vi "ImagingEventStream-SimpleFifoImage.vi"() -> ()   [LabVIEW 2017]
doc: "This example demonstrates how to use the Becker&Hickl LabVIEW wrapper VIs to acquire a single image in Fifo-Imaging mode.\nThe Event Data is interpreted and populates a 4D DecayMatrix which is then saved as SDT-file to disc.\n\ninfo@becker.hickl.com"
uses:
  SPC_Wrappers/SPC_Controls/SPCdata.ctl
  SPC_Wrappers/SPC_Controls/SPC_RatesCluster.ctl
  Example_Controls/UserInput.ctl
  SPC_Wrappers/SPC_Controls/StateCluster.ctl
  SPC_Wrappers/SPC_Controls/dither_range.ctl
  SPC_Wrappers/Initialisation/SPC_get_error_string.vi
panel:
  out "Overflow, Stop":bool
  out "DecayMatrix":u16[][][][](array[numeric])
  in  "Abort":bool
  in  "include Intensity Image":bool=TRUE
  out "SPC_StateCluster":T1
  in  "User Input":T2={"tac_range"=50.033573, "tac_gain"=2, "tac_offset"=5.0, "tac_limit_high"=89.803925, "tac_limit_low"=10.196078, "collect_time"=10.0, "sync_threshold"=-71.0, "sync_zc_level"=-5.2999988, "sync_freq_div"=1, "cfd_limit_low"=-50.0, "cfd_zc_level"=5.3000016} {"sync_freq_div" items=["1"=1, "2"=2, "4"=4]; "cfd_zc_level" min=-96 max=96 step=0.1 format="%#_3g"; "cfd_limit_low" min=-500 max=0 step=0.1 format="%#_3g"; "sync_zc_level" min=-96 max=96 step=0.1 format="%#_3g"; "sync_threshold" min=-500 max=-20 step=0.1 format="%#_3g"; "tac_limit_low" format="%.3g"; "tac_limit_high" min=0 max=100 step=0.1 format="%.3g"; "collect_time" min=1e-07 max=100000 step=0.001; "tac_offset" min=0 max=100 step=0.1 format="%.4g"; "tac_gain" min=1 max=15 step=1; "tac_range" format="%^#_6g"}
  out "Photon Count":u64
  in  "NoOfRoutingChannels":u32=1 min=1 max=128 step=1
  out "IntensityImage":u32[][](graph)
  in  "ActiveModule":i32[](listbox)
  out "Curent Read Count":u32 step=1
  in  "SDT-File Path":path=path "C:/temp/test.sdt"
  out "MT clock [ns]":i32=25
  out "AquiredPxEvents":cluster{"X":i32, "Y":i32}
  out "SumOfDecays":u32[](graph)=[0, 0, 0, 0, 0, 0, 0, 0, 0, 0, 0, 0, 0, 0, 0, 0, 0, 0, 0, 0, 0, 0, 0, 0, 0, 0, 0, 0, 0, 0, 0, 0, 0, 0, 0, 0, 0, 0, 0, 0, 0, 0, 0, 0, 0, 0, 0, 0, 0, 0, 0, 0, 0, 0, 0, 0, 0, 0, 0, 0, 0, 0, 0, 0, 0, 0, 0, 0, 0, 0, 0, 0, 0, 0, 0, 0, 0, 0, 0, 0, 0, 0, 0, 0, 0, 6, 125, 109, 110, 121, 134, 1104, 3322, 4416, 4644, 4252, 3880, 3585, 3338, 3099, 2923, 2680, 2526, 2363, 2302, 2065, 2037, 1850, 1835, 1680, 1618, 1495, 1415, 1340, 1354, 1344, 1230, 1205, 1110, 1099, 1055, 1073, 969, 897, 915, 879, 826, 828, 779, 761, 760, 741, 674, 666, 635, 675, 612, 654, 541, 599, 580, 511, 492, 520, 489, 482, 463, 436, 481, 442, 415, 420, 393, 409, 416, 362, 382, 349, 345, 338, 324, 324, 344, 328, 286, 322, 307, 275, 277, 289, 241, 289, 239, 239, 269, 257, 232, 198, 222, 228, 222, 226, 207, 188, 224, 205, 227, 178, 188, 200, 177, 158, 177, 188, 171, 179, 168, 156, 146, 163, 146, 163, 146, 123, 140, 157, 149, 116, 145, 112, 132, 122, 149, 92, 0, 0, 0, 0, 0, 0, 0, 0, 0, 0, 0, 0, 0, 0, 0, 0, 0, 0, 0, 0, 0, 0, 0, 0, 0, 0, 0, 0, 0, 0, 0, 0, 0, 0, 0, 0, 0, 0, 0, 0, 0, 0]
  out "DLL Path":path=path "C:/Program Files (x86)/BH/SPCM/DLL/spcm64.dll"
  out "Clock Status":T3={"Frame Clock"=TRUE, "Line Clock"=TRUE, "Pixel Clock"=TRUE}
  out "SPC_RatesCluster":T4 {"Sync" scale=0.0..6000000.0; "ADC" scale=0.0..1000000.0; "TAC" scale=0.0..1000000.0; "CFD" scale=0.0..1000000.0}
  out "SPCdata":T5={"base_adr"=52672, "init"=0, "cfd_limit_low"=-0.0, "cfd_limit_high"=5.019608, "cfd_zc_level"=-5.2913384, "cfd_holdoff"=5.0, "sync_zc_level"=-5.2913384, "sync_holdoff"=4.0, "sync_threshold"=-70.588234, "tac_range"=50.033573, "sync_freq_div"=1, "tac_gain"=1, "tac_offset"=5.098039, "tac_limit_low"=0.0, "tac_limit_high"=100.0, "adc_resolution"=12, "ext_latch_delay"=0, "collect_time"=1.0, "display_time"=1.0, "repeat_time"=10.0, "stop_on_time"=1, "stop_on_ovfl"=1, "dither_range"=128, "count_incr"=1, "mem_bank"=0, "dead_time_comp"=0, "scan_control"=0, "routing_mode"=0, "tac_enable_hold"=0.0, "pci_card_no"=-1, "mode"=5, "scan_size_x"=1, "scan_size_y"=1, "scan_rout_x"=1, "scan_rout_y"=1, "scan_flyback"=65537, "scan_borders"=0, "scan_polarity"=0, "pixel_clock"=1, "line_compression"=1, "trigger"=0, "pixel_time"=1e-07, "ext_pixclk_div"=1, "rate_count_time"=1.0, "macro_time_clk"=0, "add_select"=0, "test_eep"=1, "adc_zoom"=0, "img_size_x"=1, "img_size_y"=1, "img_rout_x"=1, "img_rout_y"=1, "xy_gain"=1, "master_clock"=0, "adc_sample_delay"=0, "detector_type"=1, "chan_enable"=4191231, "chan_slope"=0, "chan_spec_no"=34835, "tdc_control"=0, "tdc_offset1"=0.0, "tdc_offset2"=0.0, "tdc_offset3"=0.0, "tdc_offset4"=0.0, "tdc_offset5"=0.0, "tdc_offset6"=0.0, "cfd_th5_tdc"=0.0, "cfd_th6_tdc"=0.0, "cfd_zc5_tdc"=0.0, "cfd_zc6_tdc"=0.0, "future_reserve1"=0, "future_reserve2"=0, "future_reserve3"=0, "future_reserve4"=0} {"scan_flyback" format="%x"}
  # "This example demonstrates how to use the Becker&Hickl LabVIEW wrapper VIs to acquire a single image in Fifo-Imaging mode.\nThe Event Data is interpreted and populates a 4D DecayMatrix which is then saved as SDT-file to disc."
  # "See Tip-Strip for details"
  # "TAC / Time Range"
  # "CFD"
  # "(start)"
  # "SYNC"
  # "(stop)"
  # "range"
  # "gain"
  # "threshold(LL)"
  # "offset"
  # "limit high"
  # "limit low"
  # "zero cross(ZC)"
  # "Collection Time"
  # "(c) 2022 Becker & Hickl GmbH\n     ALL RIGHTS RESERVED."
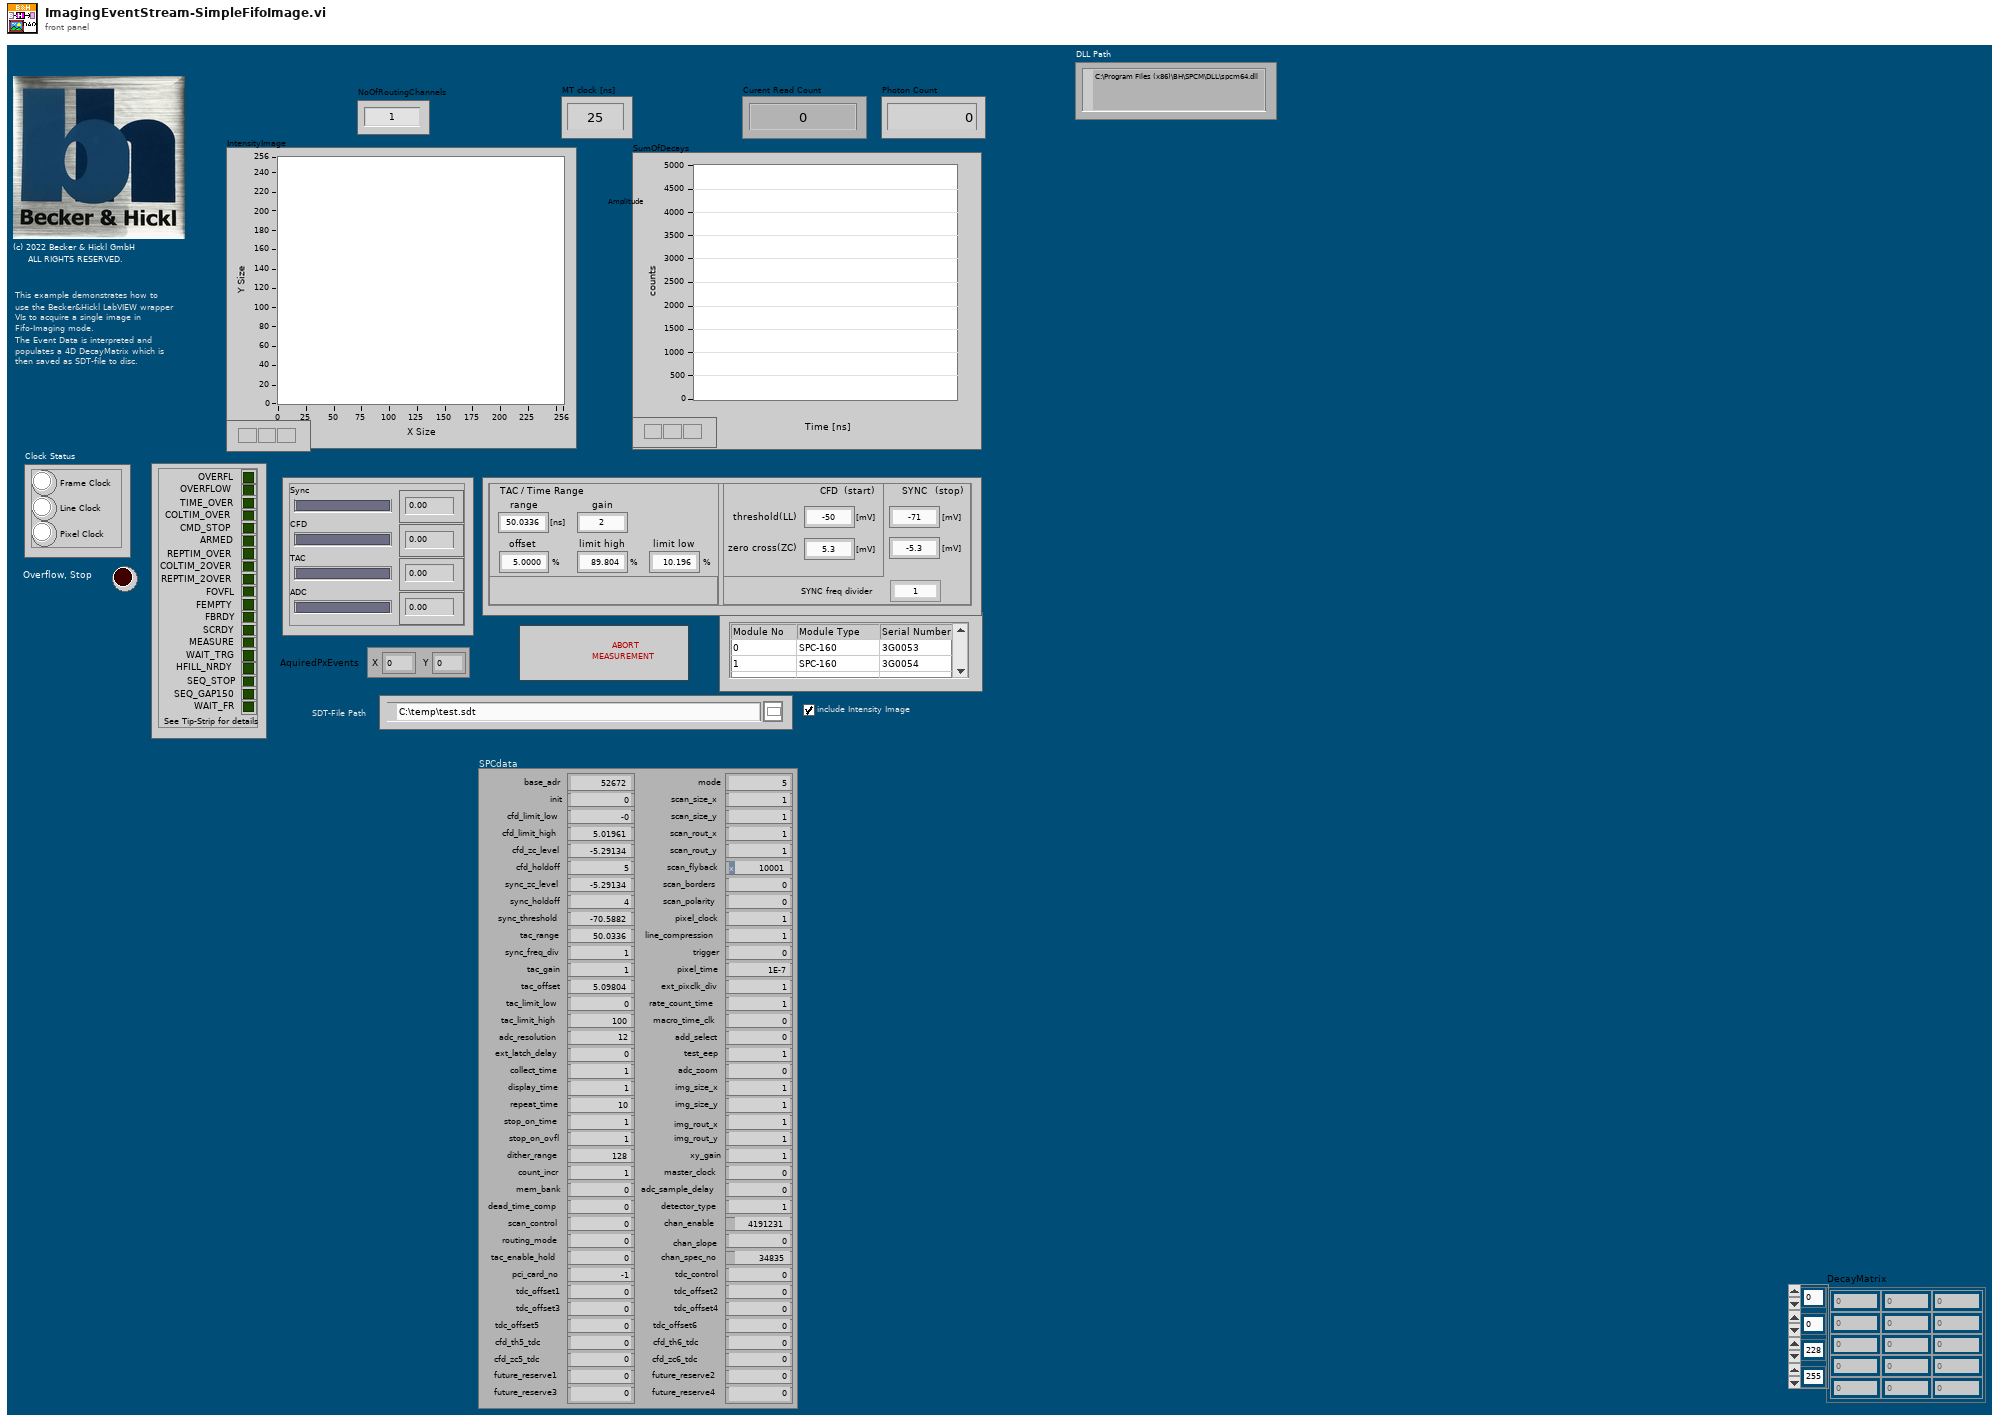
[diagram p1: front panel]
types:
  T1 = typedef "StateCluster.ctl" = cluster{"OVERFL":bool, "OVERFLOW":bool, "TIME_OVER":bool, "COLTIM_OVER":bool, "CMD_STOP":bool, "ARMED":bool, "REPTIM_OVER":bool, "COLTIM_2OVER":bool, "REPTIM_2OVER":bool, "FOVFL":bool, "FEMPTY":bool, "FBRDY":bool, "SCRDY":bool, "MEASURE":bool, "WAIT_TRG":bool, "HFILL_NRDY":bool, "SEQ_STOP":bool, "SEQ_GAP150":bool, "WAIT_FR":bool}
  T2 = typedef "UserInput.ctl" = cluster{"tac_range":sgl, "tac_gain":i16, "tac_offset":sgl, "tac_limit_high":sgl, "tac_limit_low":sgl, "collect_time":sgl, "sync_threshold":sgl, "sync_zc_level":sgl, "sync_freq_div":i16, "cfd_limit_low":sgl, "cfd_zc_level":sgl}
  T3 = cluster{"Frame Clock":bool, "Line Clock":bool, "Pixel Clock":bool}
  T4 = typedef "SPC_RatesCluster.ctl" = cluster{"Sync":sgl, "CFD":sgl, "TAC":sgl, "ADC":sgl}
  T5 = typedef "SPCdata.ctl" = cluster{"base_adr":u16, "init":i16, "cfd_limit_low":sgl, "cfd_limit_high":sgl, "cfd_zc_level":sgl, "cfd_holdoff":sgl, "sync_zc_level":sgl, "sync_holdoff":sgl, "sync_threshold":sgl, "tac_range":sgl, "sync_freq_div":i16, "tac_gain":i16, "tac_offset":sgl, "tac_limit_low":sgl, "tac_limit_high":sgl, "adc_resolution":i16, "ext_latch_delay":i16, "collect_time":sgl, "display_time":sgl, "repeat_time":sgl, "stop_on_time":i16, "stop_on_ovfl":i16, "dither_range":i16, "count_incr":i16, "mem_bank":i16, "dead_time_comp":i16, "scan_control":u16, "routing_mode":u16, "tac_enable_hold":sgl, "pci_card_no":i16, "mode":u16, "scan_size_x":u32, "scan_size_y":u32, "scan_rout_x":u32, "scan_rout_y":u32, "scan_flyback":u32, "scan_borders":u32, "scan_polarity":u16, "pixel_clock":u16, "line_compression":u16, "trigger":u16, "pixel_time":sgl, "ext_pixclk_div":u32, "rate_count_time":sgl, "macro_time_clk":i16, "add_select":i16, "test_eep":i16, "adc_zoom":i16, "img_size_x":u32, "img_size_y":u32, "img_rout_x":u32, "img_rout_y":u32, "xy_gain":i16, "master_clock":i16, "adc_sample_delay":i16, "detector_type":i16, "chan_enable":u32, "chan_slope":u32, "chan_spec_no":u32, "tdc_control":u32, "tdc_offset1":sgl, "tdc_offset2":sgl, "tdc_offset3":sgl, "tdc_offset4":sgl, "tdc_offset5":sgl, "tdc_offset6":sgl, "cfd_th5_tdc":sgl, "cfd_th6_tdc":sgl, "cfd_zc5_tdc":sgl, "cfd_zc6_tdc":sgl, "future_reserve1":u64, "future_reserve2":u64, "future_reserve3":u64, "future_reserve4":u64}
  T6 = typedef "dither_range.ctl" = i16
  T7 = cluster{"X Size":i32, "Y Size":i32, "adc_res":i32, "NoOfRoutingChannel":i32}
  T8 = typedef "SPCModInfo.ctl" = cluster{"Module Type":T9, "Bus Number":i16, "Slot Number":i16, "in Use":i16, "Init Status":i16, "Base I/O Addr":u16}
  T9 = typedef "ModuleType.ctl" = i16
  T10 = typedef "Fifo_CounterCluster.ctl" = cluster{"Pixel No":i32, "Frame No":i32, "LastPixelTime":u64, "Line No":i32, "StopFrame":bool, "StartFrame":bool, "Frame Flag":bool, "Out Of Y":bool, "MT-Overflow":bool, "Photon Count":u64, "LineLength":i32, "FrameHeight":i32, "MT-Overflow":u64, "PixelDwellTime":u32}
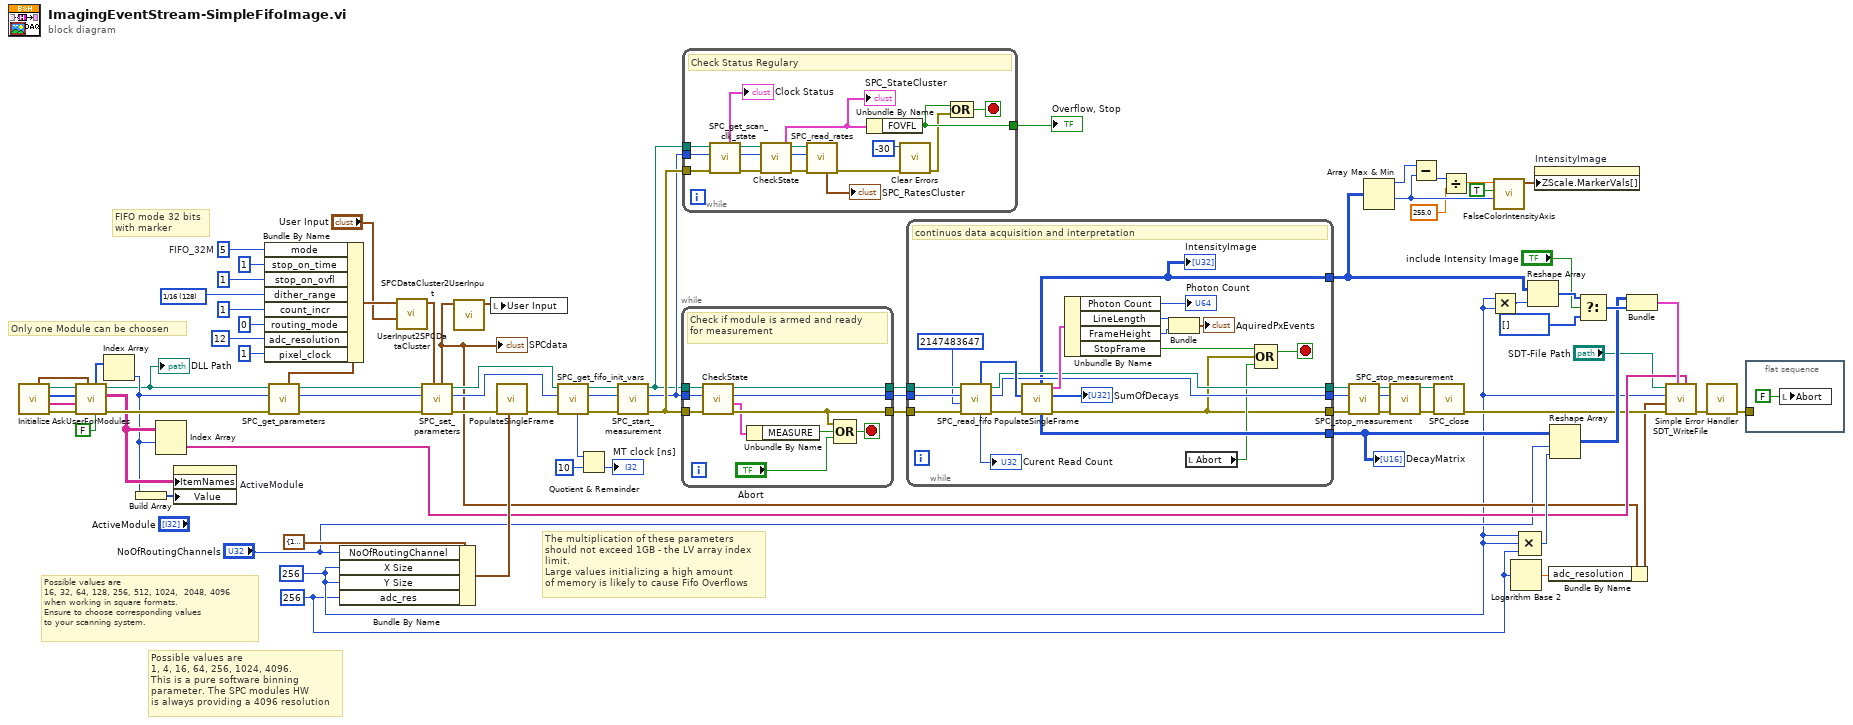
[diagram p0: block diagram]
diagram:
  w4 = T6 128 items=["0"=0, "1/64"=32, "1/32"=64, "1/16"=128, "1/8"=256] ("DithRange")
  w2 = 256 ("adc_res")
  w6 = 256 ("X Size")
  w62 = u16 5  # FIFO_32M
  # "The multiplication of these parameters \nshould not exceed 1GB - the LV array index\nlimit.\nLarge values initializing a high amount\nof memory is likely to cause Fifo Overflows"
  # "Possible values are\n1, 4, 16, 64, 256, 1024, 4096.\nThis is a pure software binning\nparameter. The SPC modules HW\nis always providing a 4096 resolution"
  # "Possible values are \n16, 32, 64, 128, 256, 512, 1024,  2048, 4096\nwhen working in square formats.\nEnsure to choose corresponding values\nto your scanning system."
  # "FIFO mode 32 bits\nwith marker"
  # "Only one Module can be choosen"
  n1 = call "Initialize.vi"() -> ("ErrorOut"=w60:errorcluster, "SerialNumbersArray"=w57:string[], "ModuleNoArray"=w59:i16[], "DLL Path"=w58:path, "SPCModulesArray"=w56:T8[])  [unwired: 7 in]
  n2 = call "AskUserForModules.vi"("MultiModule"=FALSE, "SPCModulesArray"=w56, "Error In"=w60, "Serial Number"=w57, "ModuleNoArray"=w59, "DLL Path"=w58) -> ("Error Out"=w49:errorcluster, "ModuleListboxStrings"=w33:string[][], "DLL Path"=w21:path, "ActiveModuleNo"=w61:i16[])  [unwired: 1 in, 1 out]
  "DLL Path" <- w21
  n3 = Index Array(array=w61) -> (element=w32:i16)  [unwired: 1 in]
  n4 = Build Array(w32) -> (w55:i16[])
  n5 = Index Array(array=w33, index (row)=w32) -> (element=w31:string[])  [unwired: 1 in]
  n6 = property on="ActiveModule" class="MCListbox (strict)"("ItemNames"=w33, "Value"=w55) -> ()  [unwired: 2 in, 2 out]
  n7 = call "SPC_get_parameters.vi"("Error In"=w49, "Module No"=w32, "DLL Path"=w21) -> ("Error Out"=w48:errorcluster, "Module No"=w47:i16, "DLL Path"=w46:path, "SPCdata"=w54:T5)  [unwired: 5 in]
  n8 = Bundle By Name(cluster=w54, "mode"=w62, "stop_on_time"=i16 1 ("Stop on Time"), "stop_on_ovfl"=i16 1 ("Stop on Overflow"), "dither_range"=w4, "count_incr"=i16 1 ("Count Increment"), "routing_mode"=u16 0 ("Routing Mode"), "adc_resolution"=i16 12 ("ADC Resolution"), "pixel_clock"=u16 1 ("Pixel Clock Source")) -> (w53:T5)
  n9 = Bundle By Name(cluster=T7 {"X Size"=127, "Y Size"=127, "adc_res"=127, "NoOfRoutingChannel"=1} ("Image Size"), "NoOfRoutingChannel"="NoOfRoutingChannels", "X Size"=w6, "Y Size"=w6, "adc_res"=w2) -> (w76:T7)
  n10 = call "UserInput2SPCDataCluster.vi"("UserInput_In"="User Input", "SPCData_In"=w53) -> ("SPCData_Out"=w51:T5)  [unwired: 9 in]
  n11 = call "SPC_set_parameters.vi"("SPCdata In"=w51, "Error In"=w48, "Module No."=w47, "DLL Path"=w46) -> ("Error Out"=w45:errorcluster, "Module No"=w37:i16, "DLL Path"=w36:path, "SPCdata Out"=w25:T5)  [unwired: 4 in]
  "SPCdata" <- w25
  n12 = call "SPCDataCluster2UserInput.vi"("SPCdata In"=w25) -> ("UserInput Out"=w50:T2)  [unwired: 10 in]
  n13 = local write "User Input"(w50) -> ()
  n14 = call "PopulateSingleFrame.vi"("New Image Size\nwhen != 0"=w76, "Error In"=w45) -> ("Error Out"=w38:errorcluster)  [unwired: 5 in, 4 out]
  n15 = call "SPC_get_fifo_init_vars.vi"("Error In"=w38, "Module No."=w37, "DLL Path"=w36) -> ("Error Out"=w79:errorcluster, "Module No."=w81:i16, "DLL Path"=w80:path, "mt_clock ( 0.1 ns units)"=w83:i32)  [unwired: 2 in, 3 out]
  n16 = Quotient & Remainder(x=w83, y=10) -> (floor(x/y)=→"MT clock [ns]":i32)  [unwired: 1 out]
  n17 = call "SPC_start_measurement.vi"("Error In"=w79, "Module No"=w81, "DLL Path"=w80) -> ("Error Out"=w35:errorcluster, "Module No"=w17:i16, "DLL Path"=w16:path)  [unwired: 6 in]
  n18 = while {
    tunnel: w16 -> [w93]
    tunnel: w17 -> [w92]
    tunnel: [w88] -> w19
    tunnel: [w86] -> w18
    tunnel: w35 -> [w91]
    tunnel: [w87] -> w34
    stop <- w90 stop-if-true
    # "Check if module is armed and ready\nfor measurement"
    n19 = call "CheckState.vi"("Error In"=w91, "Module No."=w92, "DLL Path"=w93) -> ("Error Out"=w87:errorcluster, "SPC_StateCluster"=w85:T1, "Module No."=w88:i16, "DLL Path"=w86:path)  [unwired: 4 in, 1 out]
    n20 = Unbundle By Name(w85) -> ("MEASURE"=w89:bool)
    n21 = Compound Arithmetic op=OR(w87, w89, "Abort") -> (w90:bool)
  }
  n22 = while {
    tunnel: [w97] -> w7
    tunnel: w35 -> [w110]
    tunnel: w17 -> [w109]
    tunnel: w16 -> [w108]
    stop <- w95 stop-if-true
    # "Check Status Regulary"
    n23 = call "SPC_get_scan_clk_state.vi"("Error In"=w110, "Module No"=w109, "DLL Path"=w108) -> ("Error Out"=w103:errorcluster, "Module No"=w99:i16, "DLL Path"=w100:path, "Clock Status"=→"Clock Status":T3)  [unwired: 4 in, 1 out]
    n24 = call "CheckState.vi"("Error In"=w103, "Module No."=w99, "DLL Path"=w100) -> ("Error Out"=w104:errorcluster, "SPC_StateCluster"=w94:T1, "Module No."=w101:i16, "DLL Path"=w102:path)  [unwired: 4 in, 1 out]
    "SPC_StateCluster" <- w94
    n25 = call "SPC_read_rates.vi"("Error In"=w104, "Module No"=w101, "DLL Path"=w102) -> ("Error Out"=w107:errorcluster, "SPC_RatesCluster"=→"SPC_RatesCluster":T4)  [unwired: 5 in, 2 out]
    n26 = Unbundle By Name(w94) -> ("FOVFL"=w97:bool)
    n27 = call <vilib>:"Clear Errors.vi"("error in (no error)"=w107, "specific error code to clear (0: all)"=-30) -> ("error out"=w96:errorcluster)  [unwired: 4 in, 1 out]
    n28 = Compound Arithmetic op=OR(w97, w96) -> (w95:bool)
  }
  "Overflow, Stop" <- w7
  n29 = while {
    tunnel: [w115] -> w30
    tunnel: [w112] -> w9
    tunnel: w18 -> [w130]
    tunnel: [w119] -> w39
    tunnel: w19 -> [w129]
    tunnel: [w118] -> w40
    tunnel: w34 -> [w131]
    tunnel: [w111] -> w41
    stop <- w114 stop-if-true
    # "continuos data acquisition and interpretation"
    n30 = call "SPC_read_fifo.vi"("Error In"=w131, "Input Count"=2147483647, "Module No"=w129, "DLL Path"=w130) -> ("Error Out"=w124:errorcluster, "Module No"=w118:i16, "DLL Path"=w119:path, "Output Count"=→"Curent Read Count":u32, "Data Buffer"=w123:u16[])  [unwired: 3 in]
    n31 = call "PopulateSingleFrame.vi"("Error In"=w124, "EventData"=w123) -> ("Error Out"=w111:errorcluster, "DecaySum"=→"SumOfDecays":u32[], "CounterCluster"=w121:T10, "DecayMatrix"=w115:u16[][][][], "IntensityGraph"=w112:u32[][])  [unwired: 5 in]
    "IntensityImage" <- w112
    n32 = Unbundle By Name(w121) -> ("Photon Count"=→"Photon Count":u64, "LineLength"=w126:i32, "FrameHeight"=w125:i32, "StopFrame"=w120:bool)
    n33 = Bundle("LineLength"=w126, "FrameHeight"=w125) -> (→"AquiredPxEvents":cluster{"LineLength":i32, "FrameHeight":i32})  [unwired: 1 in]
    n34 = local read "Abort"() -> (w113:bool)
    n35 = Compound Arithmetic op=OR(w120, w111, w113) -> (w114:bool)
  }
  "DecayMatrix" <- w30
  n36 = call "SPC_stop_measurement.vi"("Error In"=w41, "Module No"=w40, "DLL Path"=w39) -> ("Error Out"=w43:errorcluster, "Module No"=w42:i16, "DLL Path"=w44:path)  [unwired: 6 in]
  n37 = Array Max & Min(array=w9) -> (max value=w12:u32, min value=w15:u32)  [unwired: 2 out]
  n38 = call "SPC_stop_measurement.vi"("Error In"=w43, "Module No"=w42, "DLL Path"=w44) -> ("Error Out"=w29:errorcluster, "DLL Path"=w28:path)  [unwired: 6 in, 1 out]
  n39 = Subtract(x=w12, y=w15) -> (x-y=w14:u32)
  n40 = call "SPC_close.vi"("Error In"=w29, "DLL Path"=w28) -> ("Error Out"=w27:errorcluster)  [unwired: 8 in, 1 out]
  n41 = Divide(x=w14, y=255.0) -> (x/y=w13:dbl)
  n42 = Multiply(x=w6, y=w6) -> (x*y=w74:i32)
  n43 = call "FalseColorIntensityAxis.vi"("Offset"=w15, "ViewColor"=TRUE, "Scale"=w13) -> ("ZScaleMarkerVals"=w10:cluster{dbl, "Color Box":u32}[])  [unwired: 8 in]
  n44 = Logarithm Base 2(1:w2) -> (0:w1:dbl)
  n45 = Compound Arithmetic op=MULTIPLY(w6, w6, w2) -> (w73:i32)
  n46 = Reshape Array(w9, w74) -> (w72:u32[])
  n47 = property on="IntensityImage" class="IntGraph (strict)"("ZScale.MarkerVals[]"=w10) -> ()  [unwired: 2 in, 2 out]
  n48 = Bundle By Name(cluster=w25, "adc_resolution"=w1) -> (w3:T5)
  n49 = Reshape Array(w30, "NoOfRoutingChannels", w73) -> (w69:u16[][])
  n50 = Select(t=w72, s="include Intensity Image", f=u32[] []) -> (s? t:f=w70:u32[])
  n51 = Bundle("DecayMatrix"=w69, "f"=w70) -> (w71:cluster{"DecayMatrix":u16[][], "f":u32[]})  [unwired: 1 in]
  n52 = call "SDT_WriteFile.vi"("ActiveModule"=w31, "Data"=w71, "ErrorIn"=w27, "SPCdata"=w3, "ImageSize"=w6, "SDT-FilePath"="SDT-File Path") -> ("ErrorOut"=w26:errorcluster)  [unwired: 5 in]
  n53 = call <vilib>:"Simple Error Handler.vi"("error in (no error)"=w26) -> ("error out"=w23:errorcluster)  [unwired: 4 in, 4 out]
  n54 = flat-sequence {
    tunnel: w23 -> [_]
    frame #0 {
      n55 = local write "Abort"(FALSE ("Abort")) -> ()
    }
  }
